vi "RemoveNaN.vi"() -> ()   [LabVIEW 2010]
panel:
  out "Array OUT":dbl[][](array[numeric])
  in  "Array IN":dbl[][](array[numeric])
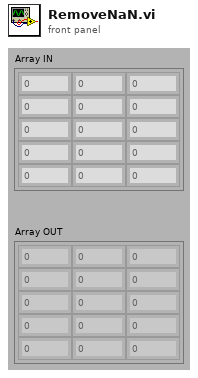
[diagram p1: front panel]
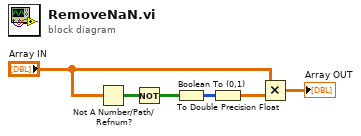
[diagram p0: block diagram]
diagram:
  n1 = Not A Number/Path/Refnum?(number/path/refnum="Array IN") -> (NaN/Path/Refnum?=w6:bool[][])
  n2 = Not(x=w6) -> (.not. x?=w5:bool[][])
  n3 = Boolean To (0,1)(Boolean=w5) -> (0, 1=w4:i16[][])
  n4 = To Double Precision Float(number=w4) -> (double precision float=w1:dbl[][])
  n5 = Multiply(x="Array IN", y=w1) -> (x*y=→"Array OUT":dbl[][])
